vi "P18_An_In.vi"() -> ()   [LabVIEW 2022 SP3]
panel:
  out "Meter":dbl(knob) scale=0.0..5.0
  out "Waveform Chart":dbl(graph)
  in  "stop":bool
  # "P18a_An_In"
  # "Equipo C\nJairo Issac García López\nRodolfo Durón Hernandez\nRoberto Carlos Herrera Pérez\nSebastián Rodríguez Posada"
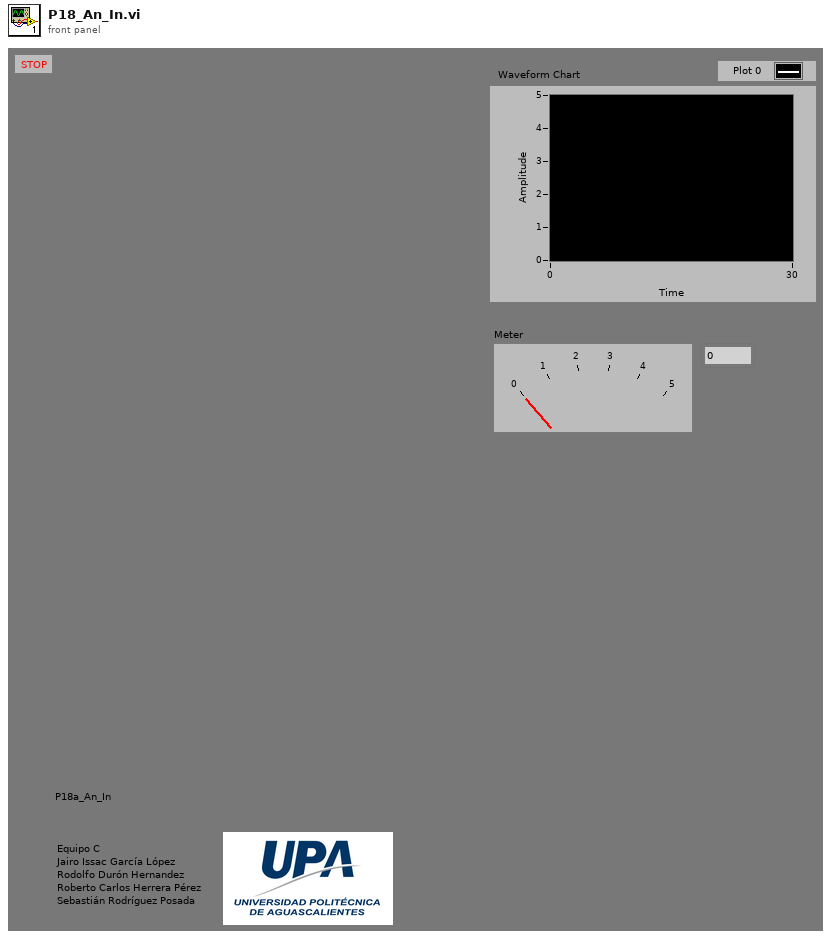
[diagram p1: front panel]
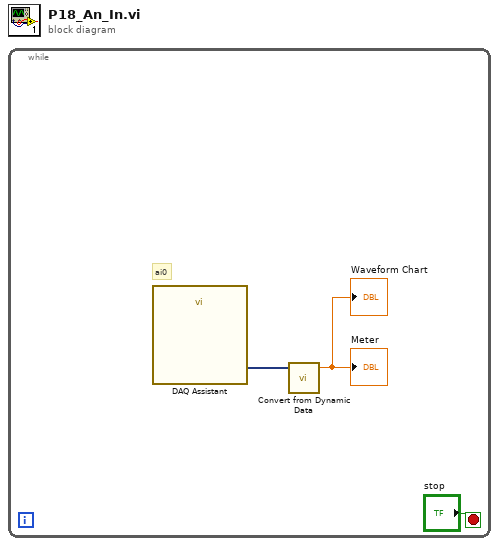
[diagram p0: block diagram]
diagram:
  n1 = while {
    stop <- "stop" stop-if-true
    # "ai0"
    n2 = call "DAQ Assistant"() -> ("data"=w2:dynamicdata)  [unwired: 17 in, 2 out]
    n3 = call "Convert from Dynamic Data"("Dynamic Data Type"=w2) -> ("Scalar"=→"Waveform Chart" →"Meter":dbl)  [unwired: 3 in]
  }
